vi "PWM UI Pins Logic.vi"(7 "Mode":enum16{"Initialize", "Process Changes"}(ring)=enum."Process Changes", 8 "error in":errorcluster, 9 "Initial Pin Names":string[](array[string]), 10 "OldVal":T1 {"Value" min=0.0 max=10.0 scale=0.0..10.0}, 11 "NewVal":T1 {"Value" min=0.0 max=10.0 scale=0.0..10.0}) -> (0 "error out":errorcluster, 3 "Updated Value":T1 {"Value" min=0.0 max=10.0 scale=0.0..10.0})   [LabVIEW 2020]
uses:
  Controls/UI-PWM Pins.ctl
  Controls/UI-PWM Pin.ctl
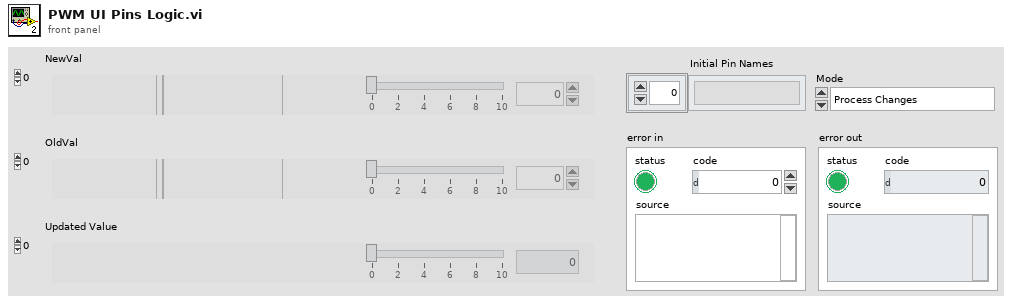
[diagram p1: front panel]
types:
  T1 = typedef "UI-PWM Pins.ctl" = T2[]
  T2 = typedef "UI-PWM Pin.ctl" = cluster{"Pin Mode":u16, "Pin Mode":string, "Value":dbl, "Pin Index":string, "Pin Modes":string}
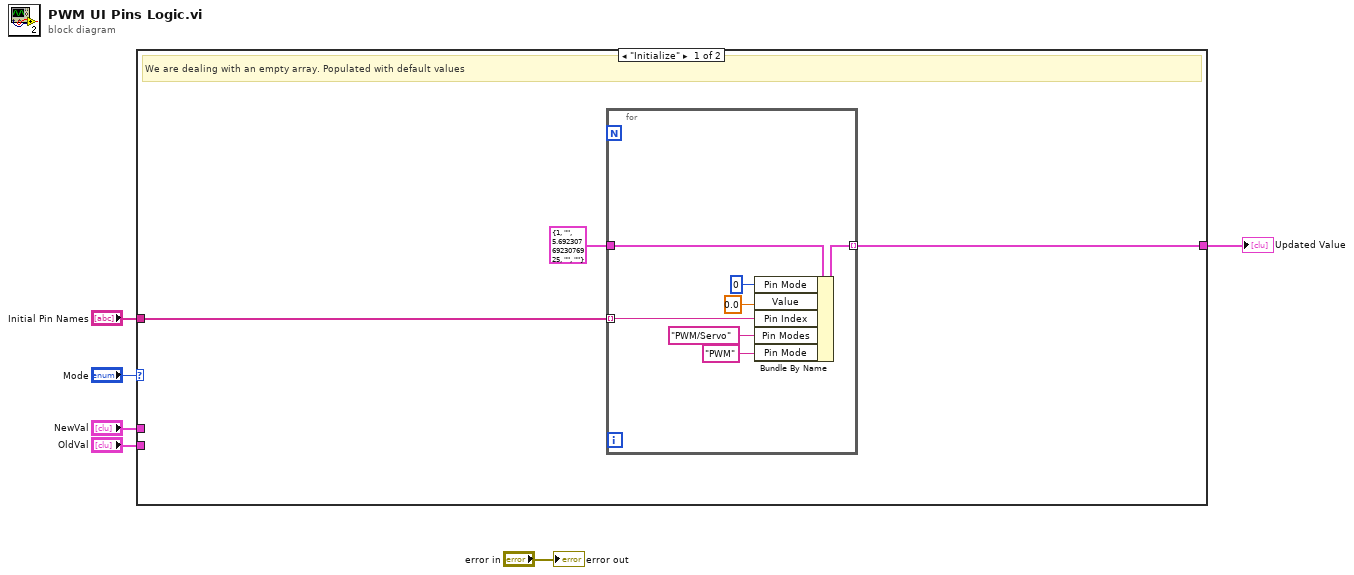
[diagram p0: block diagram]
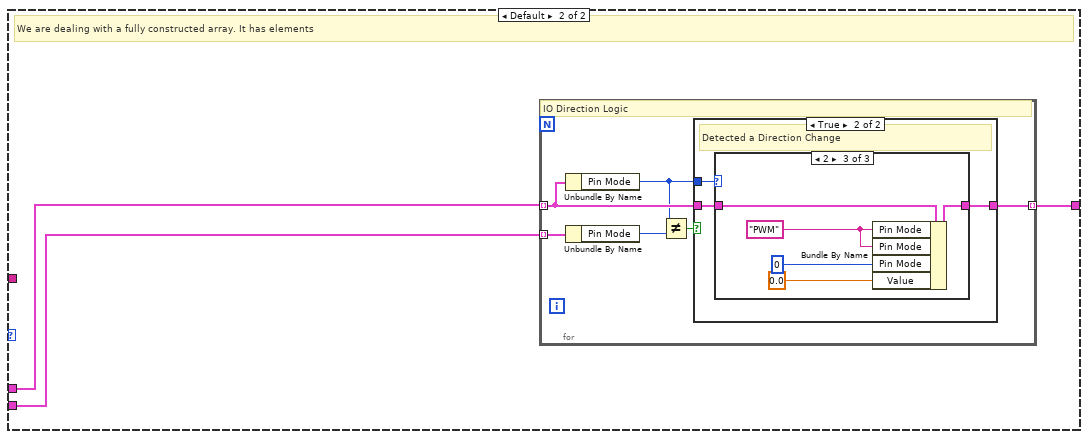
[diagram p2: hidden frame]
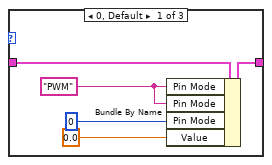
[diagram p4: hidden frame]
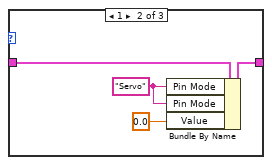
[diagram p5: hidden frame]
diagram:
  n1 = case shown="\"Initialize\"" "Mode" {
    tunnel: [w9 w19] -> w6
    tunnel: "OldVal" -> [_ w18]
    tunnel: "NewVal" -> [_ w17]
    tunnel: "Initial Pin Names" -> [w7 _]
    frame "Initialize" {
      # "We are dealing with an empty array. Populated with default values"
      n2 = for {
        tunnel: T2 {"Pin Mode"=1, "Pin Mode"="", "Value"=5.6923076923076925, "Pin Index"="", "Pin Modes"=""} ("Cluster") -> [w16]
        tunnel: [w15] -> w9 mode=indexing
        tunnel: w7 -> [w11] mode=indexing
        n3 = Bundle By Name(cluster=w16, "Pin Mode"=u16 0 ("IO Direction"), "Value"=0.0 ("AI Value"), "Pin Index"=w11, "Pin Modes"="PWM/Servo" ("Pin Mode"), "Pin Mode"="PWM" ("Pin Direction")) -> (w15:T2)
      }
    }
    frame Default {
      # "We are dealing with a fully constructed array. It has elements"
      n4 = for {
        tunnel: w17 -> [w24] mode=indexing
        tunnel: [w25] -> w19 mode=indexing
        tunnel: w18 -> [w23] mode=indexing
        # "IO Direction Logic"
        n5 = Unbundle By Name(w24) -> ("Pin Mode"=w21:u16)
        n6 = Unbundle By Name(w23) -> ("Pin Mode"=w22:u16)
        n7 = Not Equal?(x=w21, y=w22) -> (x != y?=w20:bool)
        n8 = case shown="True" w20 {
          tunnel: w21 -> [_ w29]
          tunnel: [w26 w28] -> w25
          tunnel: w24 -> [w26 w27]
          frame False {
            # "Pin has same direction"
          }
          frame True {
            # "Detected a Direction Change"
            n9 = case shown="2" w29 {
              tunnel: [w33 w37 w42] -> w28
              tunnel: w27 -> [w34 w38 w43]
              frame 0, Default {
                w30 = "PWM" ("Pin Direction")
                n10 = Bundle By Name(cluster=w34, "Pin Mode"=w30, "Pin Mode"=w30, "Pin Mode"=u16 0 ("IO Direction"), "Value"=0.0 ("Pin Value")) -> (w33:T2)
              }
              frame 1 {
                w35 = "Servo" ("Pin Direction")
                n11 = Bundle By Name(cluster=w38, "Pin Mode"=w35, "Pin Mode"=w35, "Value"=0.0 ("Pin Value")) -> (w37:T2)
              }
              frame 2 {
                w39 = "PWM" ("Pin Direction")
                n12 = Bundle By Name(cluster=w43, "Pin Mode"=w39, "Pin Mode"=w39, "Pin Mode"=u16 0 ("IO Direction"), "Value"=0.0 ("Pin Value")) -> (w42:T2)
              }
            }
          }
        }
      }
    }
  }
  "Updated Value" <- w6
  "error out" <- "error in"
